vi "Shutter Manual.vi"(8 "Error In":errorcluster, 11 "Manual Shutter in":T4) -> (0 "Error Out":errorcluster, 3 "Shutters out":T1)   [LabVIEW 2016]
uses:
  Controls/Shutter Manual.ctl
  Controls/Shutters.ctl
  Controls/Shutter Data.ctl
  Controls/Shutter States.ctl
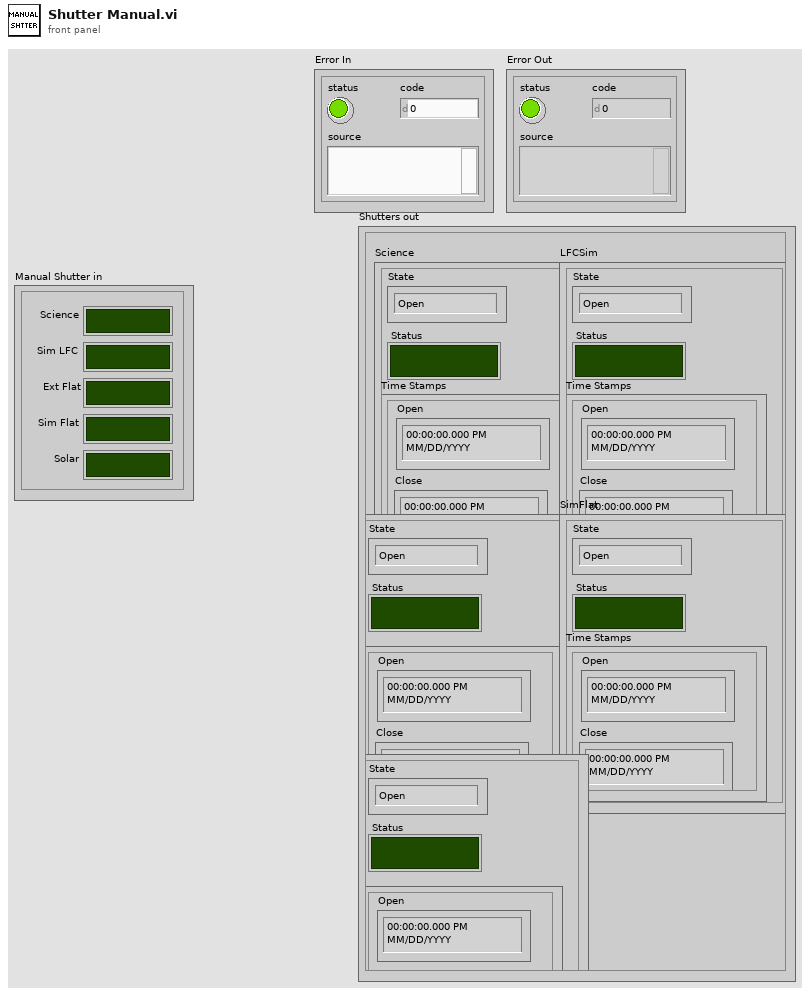
[diagram p1: front panel]
types:
  T1 = typedef "Shutters.ctl" = cluster{"Science":T2, "LFCSim":T2, "ExtendFlat":T2, "SimFlat":T2, "Solar":T2}
  T2 = typedef "Shutter Data.ctl" = cluster{"Status":bool, "State":T3, "Time Stamps":cluster{"Open":timestamp, "Close":timestamp}}
  T3 = typedef "Shutter States.ctl" = enum16{"Open", "Close", "Wait", "Off", "Arm", "Idle"}
  T4 = typedef "Shutter Manual.ctl" = cluster{"Science":bool, "Solar":bool, "Ext Flat":bool, "Sim LFC":bool, "Sim Flat":bool}
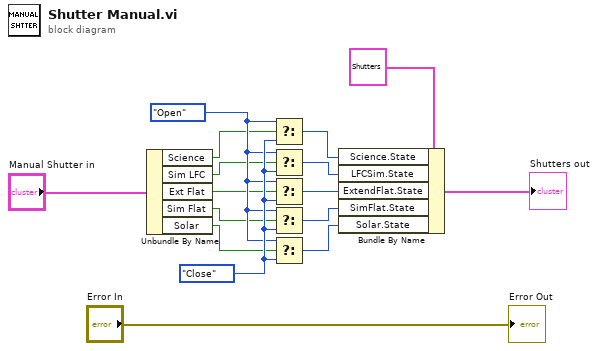
[diagram p0: block diagram]
diagram:
  w16 = Shutter_States."Close" ("Set")
  w15 = Shutter_States."Open" ("Set")
  n1 = Unbundle By Name("Manual Shutter in") -> ("Science"=w10:bool, "Sim LFC"=w11:bool, "Ext Flat"=w12:bool, "Sim Flat"=w13:bool, "Solar"=w14:bool)
  n2 = Select(t=w15, s=w10, f=w16) -> (s? t:f=w1:T3)
  n3 = Select(t=w15, s=w11, f=w16) -> (s? t:f=w5:T3)
  n4 = Select(t=w15, s=w12, f=w16) -> (s? t:f=w6:T3)
  n5 = Select(t=w15, s=w13, f=w16) -> (s? t:f=w7:T3)
  n6 = Select(t=w15, s=w14, f=w16) -> (s? t:f=w8:T3)
  n7 = Bundle By Name(cluster=T1 {"Science"={"Status"=FALSE, "State"=enum."Open", "Time Stamps"={"Open"=timestamp(0 s since 1904-01-01), "Close"=timestamp(0 s since 1904-01-01)}}, "LFCSim"={"Status"=FALSE, "State"=enum."Open", "Time Stamps"={"Open"=timestamp(0 s since 1904-01-01), "Close"=timestamp(0 s since 1904-01-01)}}, "ExtendFlat"={"Status"=FALSE, "State"=enum."Open", "Time Stamps"={"Open"=timestamp(0 s since 1904-01-01), "Close"=timestamp(0 s since 1904-01-01)}}, "SimFlat"={"Status"=FALSE, "State"=enum."Open", "Time Stamps"={"Open"=timestamp(0 s since 1904-01-01), "Close"=timestamp(0 s since 1904-01-01)}}, "Solar"={"Status"=FALSE, "State"=enum."Open", "Time Stamps"={"Open"=timestamp(0 s since 1904-01-01), "Close"=timestamp(0 s since 1904-01-01)}}} ("Shutters"), "Science.State"=w1, "LFCSim.State"=w5, "ExtendFlat.State"=w6, "SimFlat.State"=w7, "Solar.State"=w8) -> (→"Shutters out":T1)
  "Error Out" <- "Error In"
